vi "UI_History1.vi"() -> ()   [LabVIEW 2014]
panel:
  out "结果":u32
  in  "查询":bool
  in  "选项卡控件":enum32{"陪试轴承单元", "试验轴承单元", "加载单元", "主轴监测单元"}(tab)
  out "出油温度2":cluster{"X":dbl, "Y":dbl}[](graph)
  out "出油温度1":cluster{"X":dbl, "Y":dbl}[](graph)
  out "摩擦力矩":cluster{"X":dbl, "Y":dbl}[](graph)
  out "出油温度":cluster{"X":dbl, "Y":dbl}[](graph)
  out "轴承外圈温度":cluster{"X":dbl, "Y":dbl}[](graph)
  out "外壳振动2":cluster{"时间":timestamp[], "数据":dbl[]}(graph)
  out "外壳振动1":cluster{"时间":timestamp[], "数据":dbl[]}(graph)
  out "轴向油缸力":cluster{"X":dbl, "Y":dbl}[](graph)
  out "径向油缸力":cluster{"X":dbl, "Y":dbl}[](graph)
  out "径向位移SRR2":cluster{"时间":timestamp[], "数据":dbl[]}(graph)
  out "径向位移SRR1":cluster{"时间":timestamp[], "数据":dbl[]}(graph)
  out "径向位移SLR2":cluster{"时间":timestamp[], "数据":dbl[]}(graph)
  out "径向位移SLR1":cluster{"时间":timestamp[], "数据":dbl[]}(graph)
  out "轴向位移SA":cluster{timestamp[], "添加的数组":dbl[]}(graph)
  out "转速":cluster{"X":dbl, "Y":dbl}[](graph)
  in  "下拉列表":u16(ring) items=["陪试轴承单元", "试验轴承单元", "加载单元", "主轴监测单元"]
  in  "结束时间":timestamp
  in  "开始时间":timestamp
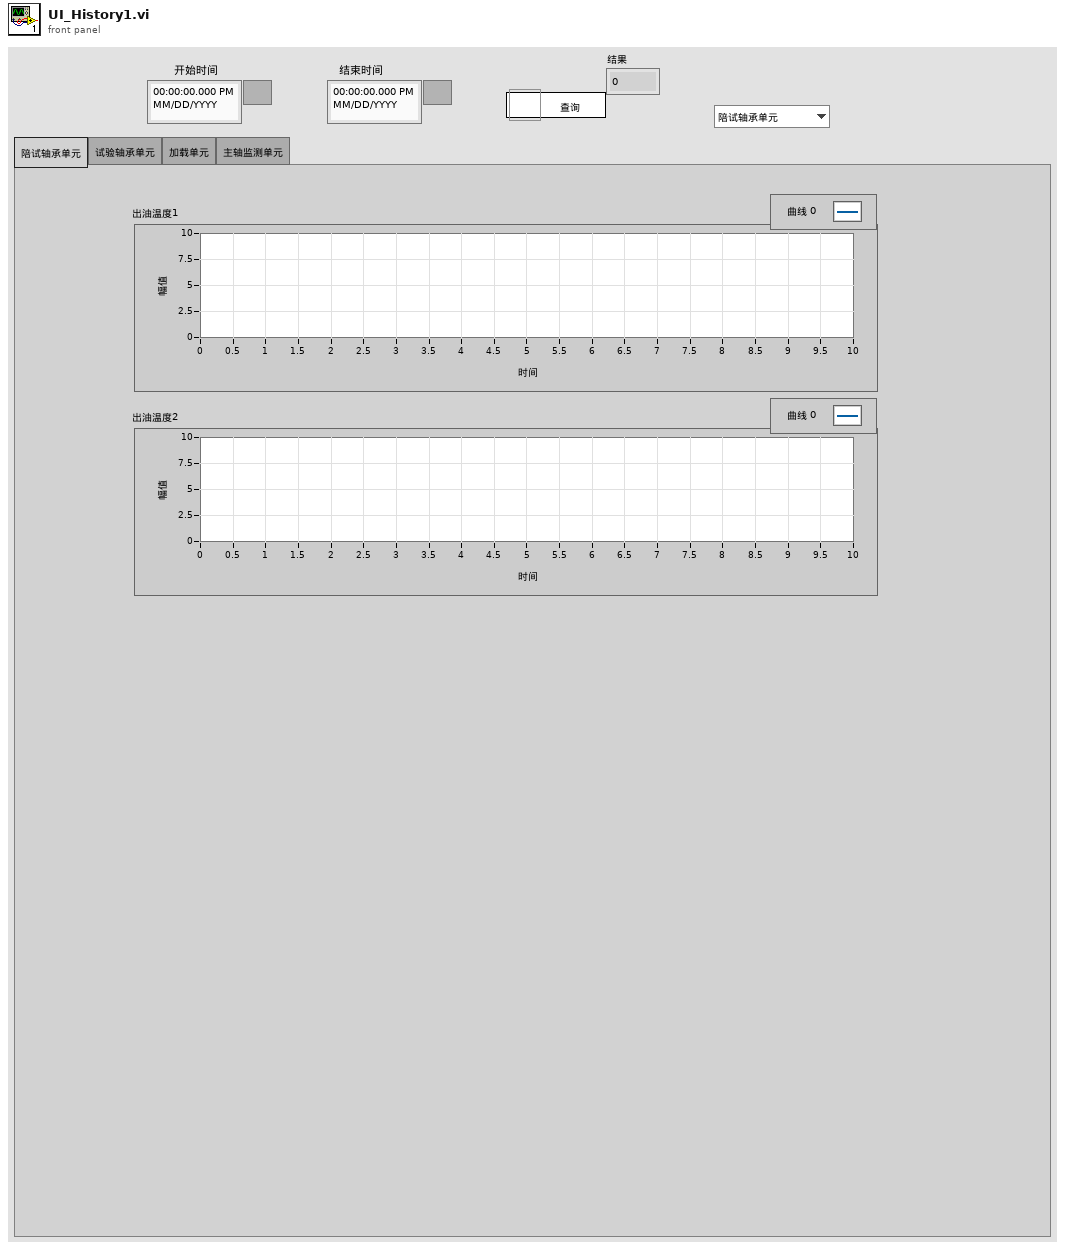
[diagram p1: front panel]
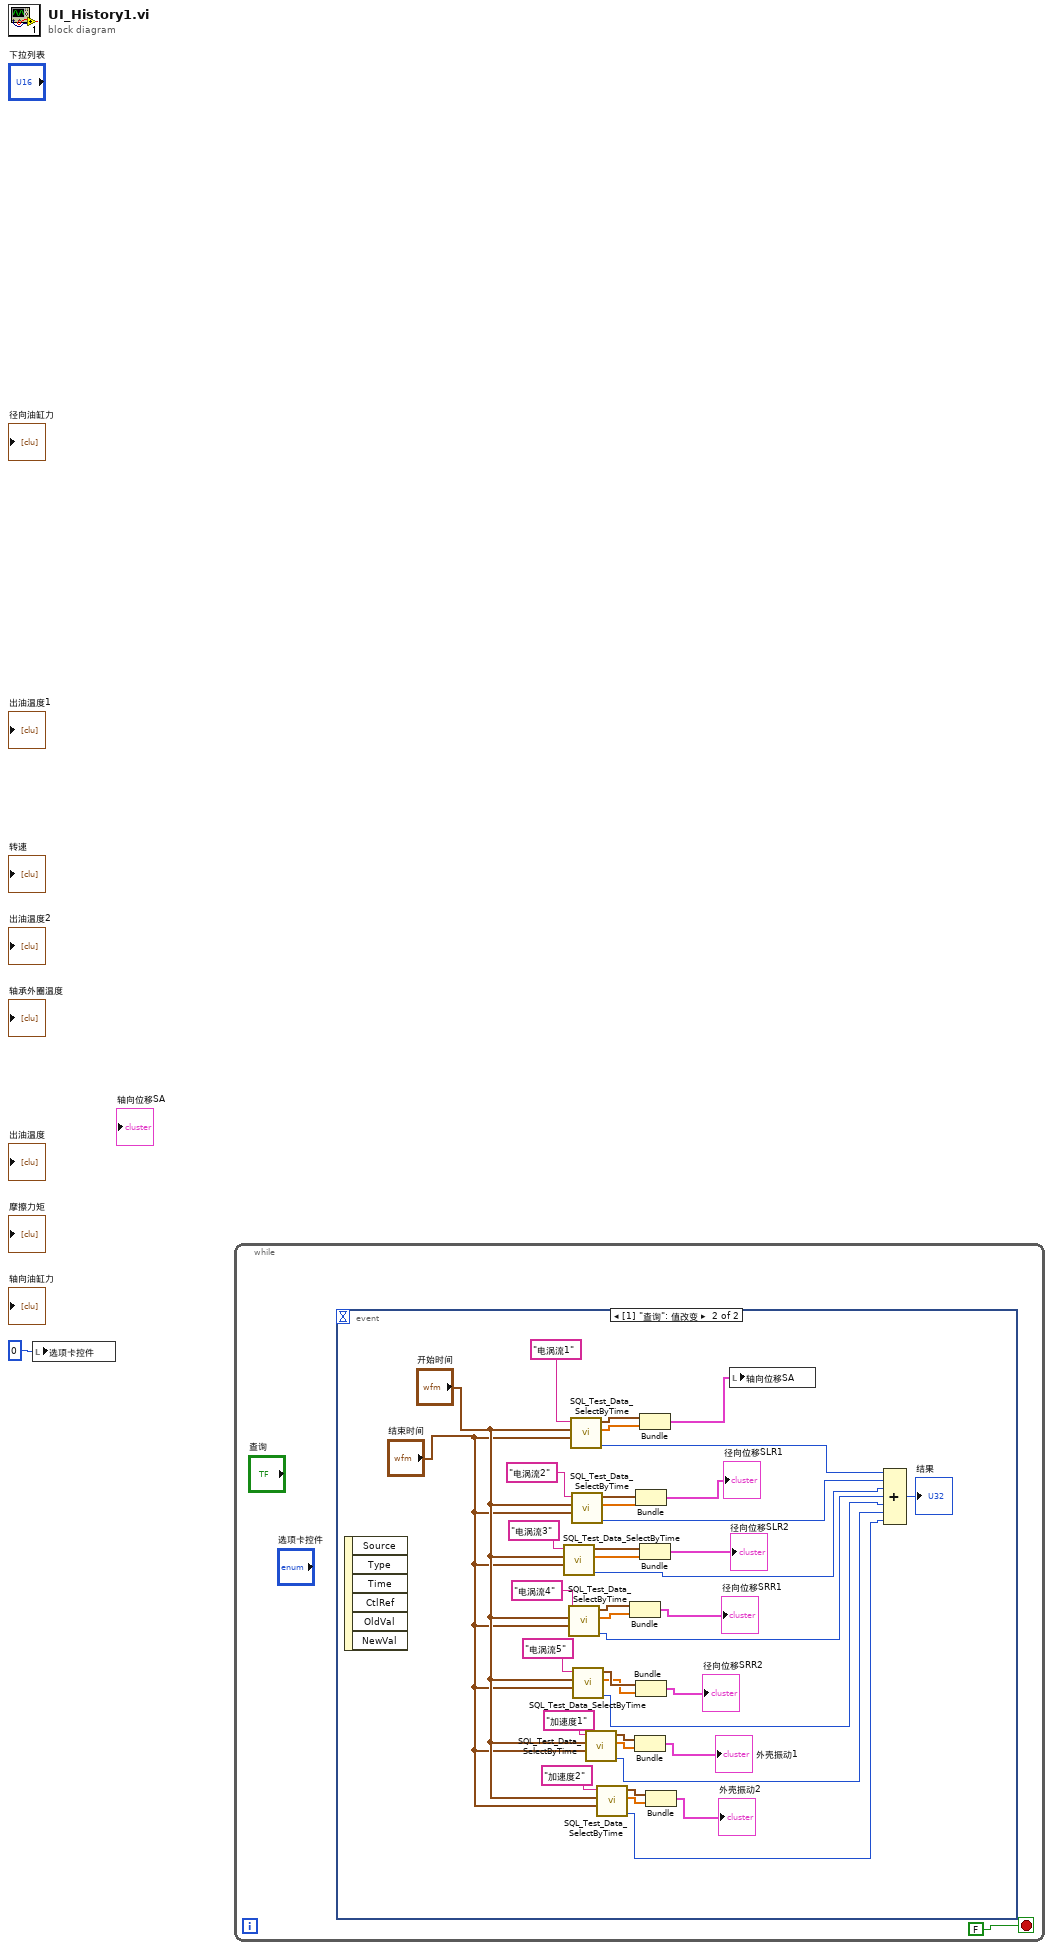
[diagram p0: block diagram]
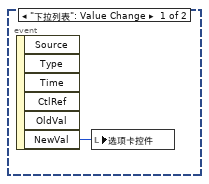
[diagram p2: hidden frame]
diagram:
  n1 = local write "选项卡控件"(0) -> ()
  n2 = while {
    stop <- FALSE stop-if-true
    n3 = event shown="[1] \"查询\": 值改变" {
      selector: _ -> [_ _]
      dyn-events: _ -> [_ _]
      timeout: _ -> [_ _]
      event "下拉列表": Value Change {
        n4 = event-data() -> ("NewVal"=w3:u16)  [unwired: 1 in, 5 out]
        n5 = local write "选项卡控件"(w3) -> ()
      }
      event "查询": Value Change {
        n6 = event-data() -> ()  [unwired: 1 in, 6 out]
        n7 = call "SQL_Test_Data_SelectByTime.vi"("结束时间"="结束时间", "起始时间"="开始时间", "通道名"="电涡流3") -> ("x-y"=w10:u32, "数据"=w32:dbl[], "时间"=w31:timestamp[])  [unwired: 3 in, 1 out]
        n8 = call "SQL_Test_Data_SelectByTime.vi"("结束时间"="结束时间", "起始时间"="开始时间", "通道名"="电涡流4") -> ("x-y"=w9:u32, "数据"=w4:dbl[], "时间"=w28:timestamp[])  [unwired: 3 in, 1 out]
        n9 = call "SQL_Test_Data_SelectByTime.vi"("结束时间"="结束时间", "起始时间"="开始时间", "通道名"="电涡流1") -> ("x-y"=w12:u32, "数据"=w39:dbl[], "时间"=w38:timestamp[])  [unwired: 3 in, 1 out]
        n10 = call "SQL_Test_Data_SelectByTime.vi"("结束时间"="结束时间", "起始时间"="开始时间", "通道名"="电涡流2") -> ("x-y"=w11:u32, "数据"=w35:dbl[], "时间"=w36:timestamp[])  [unwired: 3 in, 1 out]
        n11 = call "SQL_Test_Data_SelectByTime.vi"("结束时间"="结束时间", "起始时间"="开始时间", "通道名"="电涡流5") -> ("x-y"=w8:u32, "数据"=w25:dbl[], "时间"=w26:timestamp[])  [unwired: 3 in, 1 out]
        n12 = call "SQL_Test_Data_SelectByTime.vi"("结束时间"="结束时间", "起始时间"="开始时间", "通道名"="加速度1") -> ("x-y"=w7:u32, "数据"=w20:dbl[], "时间"=w21:timestamp[])  [unwired: 3 in, 1 out]
        n13 = call "SQL_Test_Data_SelectByTime.vi"("结束时间"="结束时间", "起始时间"="开始时间", "通道名"="加速度2") -> ("x-y"=w6:u32, "数据"=w17:dbl[], "时间"=w18:timestamp[])  [unwired: 3 in, 1 out]
        n14 = Bundle("时间"=w28, "数据"=w4) -> (→"径向位移SRR1":cluster{"时间":timestamp[], "数据":dbl[]})  [unwired: 1 in]
        n15 = Bundle("时间"=w21, "数据"=w20) -> (→"外壳振动1":cluster{"时间":timestamp[], "数据":dbl[]})  [unwired: 1 in]
        n16 = Bundle("时间"=w36, "数据"=w35) -> (→"径向位移SLR1":cluster{"时间":timestamp[], "数据":dbl[]})  [unwired: 1 in]
        n17 = Bundle("时间"=w26, "数据"=w25) -> (→"径向位移SRR2":cluster{"时间":timestamp[], "数据":dbl[]})  [unwired: 1 in]
        n18 = Bundle("时间"=w38, "数据"=w39) -> (w37:cluster{"时间":timestamp[], "数据":dbl[]})  [unwired: 1 in]
        n19 = Bundle("时间"=w31, "数据"=w32) -> (→"径向位移SLR2":cluster{"时间":timestamp[], "数据":dbl[]})  [unwired: 1 in]
        n20 = Bundle("时间"=w18, "数据"=w17) -> (→"外壳振动2":cluster{"时间":timestamp[], "数据":dbl[]})  [unwired: 1 in]
        n21 = local write "轴向位移SA"(w37) -> ()
        n22 = Compound Arithmetic op=ADD(w12, w11, w10, w9, w8, w7, w6) -> (→"结果":u32)
      }
    }
  }
